vi "Delete All SPC Parameters Files.vi"(8 "error in (no error)":errorcluster) -> (0 "error out":errorcluster)   [LabVIEW 2016]
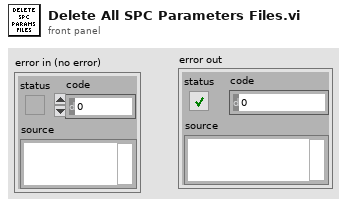
[diagram p1: front panel]
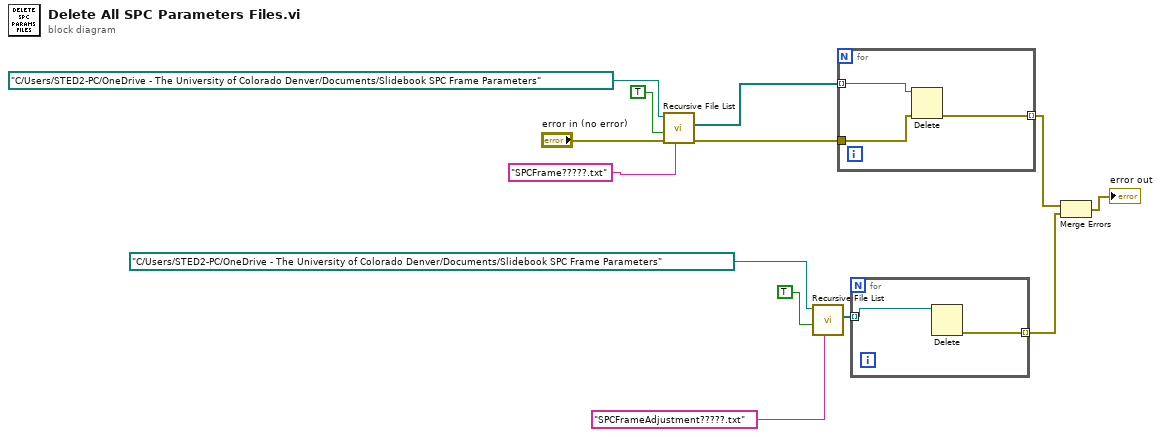
[diagram p0: block diagram]
diagram:
  n1 = call <vilib>:"Recursive File List.vi"("pattern"="SPCFrame?????.txt", "error in (no error)"="error in (no error)", "Continue Recursing on Error? (F)"=TRUE, "Folder Path"=path "C:/Users/STED2-PC/OneDrive - The University of Colorado Denver/Documents/Slidebook SPC Frame Parameters") -> ("error out"=w4:errorcluster, "All Files in Dir"=w6:path[])  [unwired: 3 in, 3 out]
  n2 = call <vilib>:"Recursive File List.vi"("pattern"="SPCFrameAdjustment?????.txt", "Continue Recursing on Error? (F)"=TRUE, "Folder Path"=path "C:/Users/STED2-PC/OneDrive - The University of Colorado Denver/Documents/Slidebook SPC Frame Parameters") -> ("All Files in Dir"=w5:path[])  [unwired: 4 in, 4 out]
  n3 = for {
    tunnel: w6 -> [w16] mode=indexing
    tunnel: [w15] -> w3 mode=indexing
    tunnel: w4 -> [w14]
    n4 = Delete(path (use dialog)=w16, error in=w14) -> (error out=w15:errorcluster)  [unwired: 3 in, 2 out]
  }
  n5 = for {
    tunnel: w5 -> [w18] mode=indexing
    tunnel: [w17] -> w2 mode=indexing
    n6 = Delete(path (use dialog)=w18) -> (error out=w17:errorcluster)  [unwired: 4 in, 2 out]
  }
  n7 = Merge Errors(w3, w2) -> (→"error out":errorcluster)
